vi "Parse Config File.vi"(8 "error in":errorcluster, 11 "XML Path":path caption="Path to XML document") -> (0 "error out":errorcluster, 3 "Custom Device Config":refnum<class "Custom Device Config.lvclass">)   [LabVIEW 2024, in "Parser.lvlib"]
uses:
  Parser.lvlib
  Custom Device Config/Custom Device Config.lvclass
  <vilib>/xml/Load XML File.vi
  <vilib>/xml/Close Reference(Node).vi
  <vilib>/xml/NI_XML.lvlib
  <resource>/objmgr/DOMUserDefRef.rc
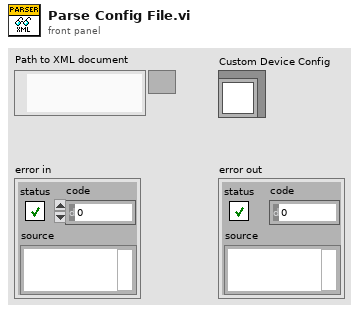
[diagram p1: front panel]
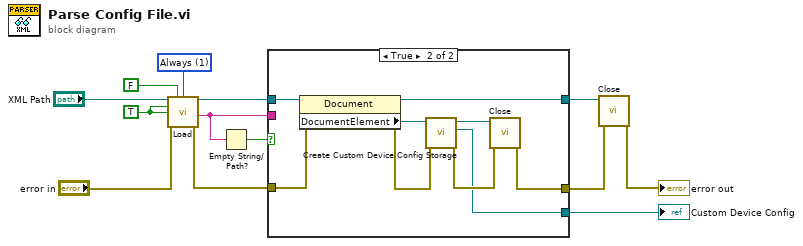
[diagram p0: block diagram]
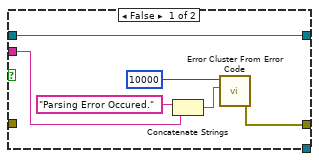
[diagram p2: hidden frame]
diagram:
  w6 = 1 items=["Never", "Always", "Auto"] ("Validate On Load")
  w7 = TRUE ("Do Namespaces")
  n1 = call-poly <vilib>:"Load.vi"("path to XML document"="XML Path", "preserve whitespace (True)"=FALSE, "validate on load (Auto)"=w6, "process namespaces (False)"=w7, "process schema (False)"=w7, "error in (no error)"="error in") -> ("DOM document out"=w4:refnum<k20>, "parse errors"=w3:string, "error out"=w11:errorcluster)  [unwired: 1 in, 6 out]
  n2 = Empty String/Path?(string/path=w3) -> (empty?=w8:bool)
  n3 = case shown="True" w8 {
    tunnel: w11 -> [_ w28]
    tunnel: w4 -> [w14 w24]
    tunnel: [w14 w23] -> w9
    tunnel: [w19 w25] -> w12
    tunnel: w3 -> [w17 _]
    tunnel: [_ w20] -> w1
    frame False {
      n4 = Concatenate Strings("Parsing Error Occured." ("error message (\"\")"), w17) -> (w15:string)
      n5 = call <vilib>:"Error Cluster From Error Code.vi"("error message (\"\")"=w15, "error code (0)"=10000) -> ("error out"=w19:errorcluster)  [unwired: 7 in]
    }
    frame True {
      n6 = property on="Property Node" class="Document"(reference=w24, error in=w28) -> (reference out=w23:refnum<k20>, error out=w27:errorcluster, "DocumentElement"=w22:refnum<k20>)
      n7 = call "Create Custom Device Config Storage.vi"("error in"=w27, "Document Element"=w22) -> ("error out"=w26:errorcluster, "Custom Device Config out"=w20:refnum<class "Custom Device Config.lvclass">, "Document Element"=w21:refnum<k20>)  [unwired: 7 in]
      n8 = call-poly <vilib>:"Close.vi"("error in (no error)"=w26, "node"=w21) -> ("error out"=w25:errorcluster)  [unwired: 7 in]
    }
  }
  "Custom Device Config" <- w1
  n9 = call-poly <vilib>:"Close.vi"("error in (no error)"=w12, "node"=w9) -> ("error out"=→"error out":errorcluster)  [unwired: 7 in]
